vi "Get Measurement Names.vi"(11 "error in (no error)":errorcluster) -> (4 "Build Details":T1[](array[typedef]), 15 "error out":errorcluster)   [LabVIEW 2021, in "Measurement Builder.lvlib"]
uses:
  Measurement Builder.lvlib
  controls/Build Spec Details.ctl
  <vilib>/AppBuilder/AB_API/common/AB_API Build Object Selector.ctl
  <vilib>/AppBuilder/AB_API/Build/NI_AB_API_Build.lvclass
  Dictionary/Dictionary.lvlib
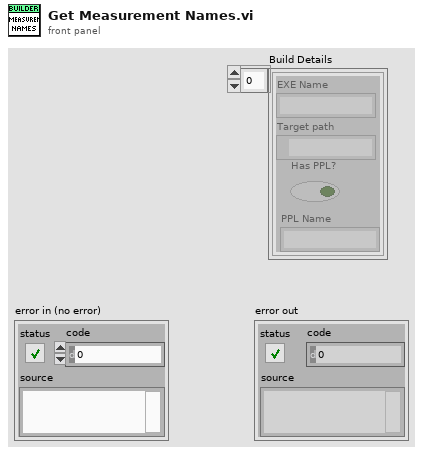
[diagram p1: front panel]
types:
  T1 = typedef "Measurement Builder.lvlib/Build Spec Details.ctl" = cluster{"EXE Name":string, "Target path":path, "Has PPL?":bool, "PPL Name":string}
  T2 = typedef "AB_API Build Object Selector.ctl" = enum16{"Source Distribution", "Deployable Source Distribution", "DLL", "EXE", "Packed Library", "Deployable Packed Library", "RT EXE", ".NET Interop Assembly"}
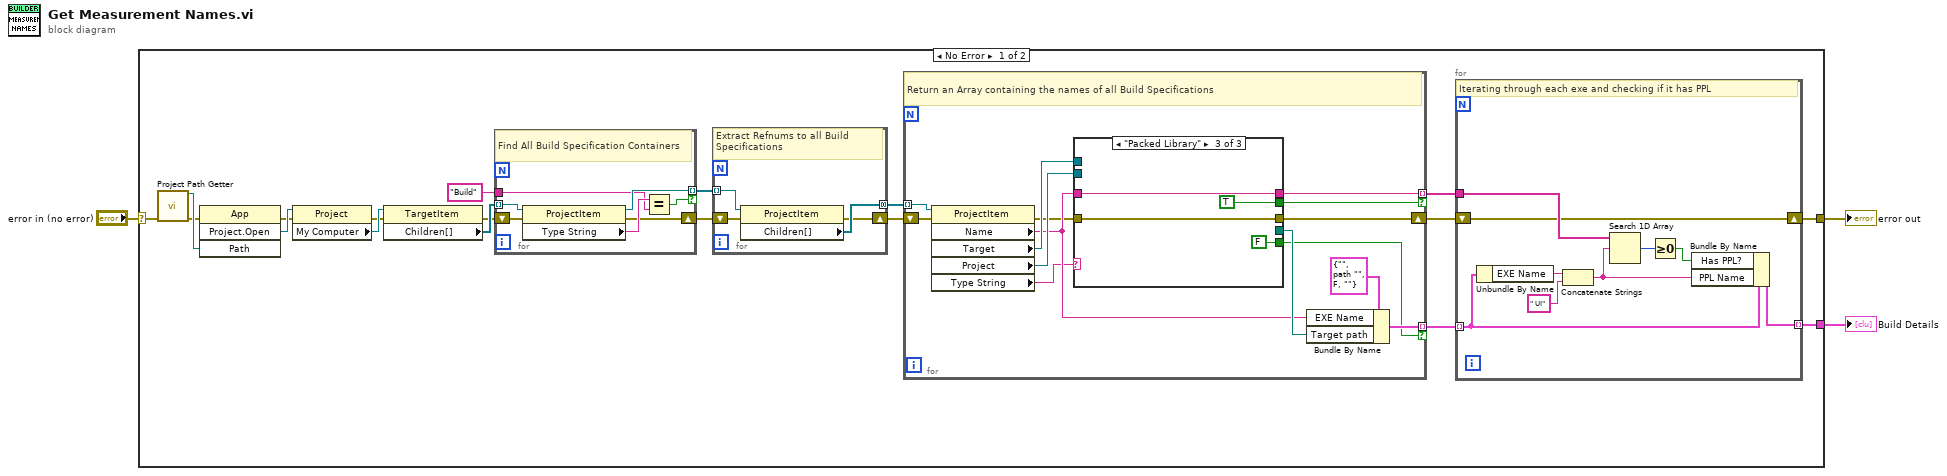
[diagram p0: block diagram]
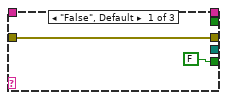
[diagram p2: hidden frame]
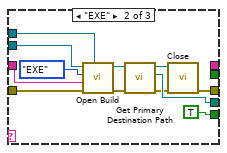
[diagram p3: hidden frame]
diagram:
  n1 = case shown="No Error" "error in (no error)" {
    selector: "error in (no error)" -> [w18 w75]
    tunnel: [w7 w75] -> w2
    tunnel: [w6 _] -> w1
    frame No Error {
      n2 = call "Project Path Getter.vi"("error in (no error)"=w18) -> ("Path"=w5:path, "error out"=w4:errorcluster)  [unwired: 13 in]
      n3 = invoke class="App" method="Project.Open"(error in=w4, "Path"=w5) -> (error out=w14:errorcluster, "Project:Open"=w16:refnum<vi>)  [unwired: 2 in, 2 out]
      n4 = property class="Project"(reference=w16, error in=w14) -> (error out=w13:errorcluster, "My Computer"=w15:refnum<vi>)  [unwired: 1 out]
      n5 = property class="TargetItem"(reference=w15, error in=w13) -> (error out=w17:errorcluster, "Children[]"=w20:refnum<vi>[])  [unwired: 1 out]
      n6 = for {
        tunnel: w20 -> [w65] mode=indexing
        tunnel: [w63] -> w21 mode=indexing if=w62
        tunnel: "Build" ("y") -> [w61]
        shift-right: [w59] -> w12
        shift-left: w17 -> [w60]
        # "Find All Build Specification Containers"
        n7 = property class="ProjectItem"(reference=w65, error in=w60) -> (reference out=w63:refnum<vi>, error out=w59:errorcluster, "Type String"=w64:string)
        n8 = Equal?(x=w64, y=w61) -> (x = y?=w62:bool)
      }
      n9 = for {
        tunnel: w21 -> [w58] mode=indexing
        tunnel: [w57] -> w19 mode=concatenating
        shift-right: [w55] -> w11
        shift-left: w12 -> [w56]
        # "Extract Refnums to all Build Specifications"
        n10 = property class="ProjectItem"(reference=w58, error in=w56) -> (error out=w55:errorcluster, "Children[]"=w57:refnum<vi>[])  [unwired: 1 out]
      }
      n11 = for {
        tunnel: w19 -> [w32] mode=indexing
        shift-right: [w27] -> w10
        shift-left: w11 -> [w31]
        tunnel: [w30] -> w9 mode=indexing if=w29
        tunnel: [w25] -> w8 mode=indexing if=w24
        # "Return an Array containing the names of all Build Specifications"
        n12 = property class="ProjectItem"(reference=w32, error in=w31) -> (error out=w28:errorcluster, "Name"=w33:string, "Target"=w34:refnum<vi>, "Project"=w35:refnum<vi>, "Type String"=w26:string)  [unwired: 1 out]
        n13 = case shown="\"Packed Library\"" w26 {
          tunnel: [_ w50 _] -> w36
          tunnel: w35 -> [_ w46 _]
          tunnel: w34 -> [_ w45 _]
          tunnel: w33 -> [_ w43 w52]
          tunnel: [FALSE TRUE FALSE] -> w29
          tunnel: w28 -> [w37 w40 w54]
          tunnel: [w37 w39 w54] -> w27
          tunnel: [_ _ w52] -> w25
          tunnel: [_ _ TRUE] -> w24
          frame "False", Default {
          }
          frame "EXE" {
            n14 = call <vilib>:"Open Build.vi"("TargetItem Refnum"=w45, "error in (no error)"=w40, "Build specification name"=w43, "Build object selector"=AB_API_Build_Object_Selector."EXE", "Project Refnum"=w46) -> ("error out"=w42:errorcluster, "NI_AB_API_Build out"=w47:refnum<class "NI_AB_API_Build.lvclass">)  [unwired: 5 in]
            n15 = call-dynamic "Get Primary Destination Path.vi"("error in (no error)"=w42, "NI_AB_API_Build in"=w47) -> ("error out"=w49:errorcluster, "Primary destination path"=w50:path, "NI_AB_API_Build out"=w48:refnum<class "NI_AB_API_Build.lvclass">)  [unwired: 7 in]
            n16 = call-dynamic "Close.vi"("error in (no error)"=w49, "NI_AB_API_Build in"=w48) -> ("error out"=w39:errorcluster)  [unwired: 9 in]
          }
          frame "Packed Library" {
          }
        }
        n17 = Bundle By Name(cluster=T1 {"EXE Name"="", "Target path"=path "", "Has PPL?"=FALSE, "PPL Name"=""}, "EXE Name"=w33, "Target path"=w36) -> (w30:T1)
      }
      n18 = for {
        tunnel: w9 -> [w70] mode=indexing
        tunnel: w8 -> [w72]
        tunnel: [w67] -> w6 mode=indexing
        shift-right: [w66] -> w7
        shift-left: w10 -> [w66]
        # "Iterating through each exe and checking if it has PPL"
        n19 = Unbundle By Name(w70) -> ("EXE Name"=w74:string)
        n20 = Concatenate Strings(w74, " UI" ("string")) -> (w68:string)
        n21 = Search 1D Array(1D array=w72, element=w68) -> (index of element=w71:i32)  [unwired: 1 in]
        n22 = Greater Or Equal To 0?(x=w71) -> (x >= 0?=w69:bool)
        n23 = Bundle By Name(cluster=w70, "Has PPL?"=w69, "PPL Name"=w68) -> (w67:T1)
      }
    }
    frame Error {
    }
  }
  "error out" <- w2
  "Build Details" <- w1
